vi "GeneratePointsForStage.vi"(8 "error in (no error)":errorcluster, 10 "Point Spacing":i32=20, 11 "Rotated Rect":T1(array[cluster])) -> (0 "error out":errorcluster, 3 "PointsInRotatedRect":cluster{"X":i32, "Y":i32}[](array[cluster]))   [LabVIEW 2017]
doc: "Use this template to build a VI to use as a subVI."
uses:
  <vilib>/Analysis/geometry.llb/Point in Polygon Position.ctl
  <vilib>/Analysis/coordinate.llb/2D Cartesian Coordinate Shift (Array).vi
  <vilib>/Analysis/coordinate.llb/2D Cartesian Coordinate Rotation (Array).vi
  <vilib>/Analysis/geometry.llb/Point in Polygon (Scalar).vi
  <vilib>/Analysis/NI_AAL_Geometry.lvlib
  <vilib>/Analysis/NI_AALPro.lvlib
panel:
  out "point":cluster{"x":i16, "y":i16}={"x"=1139, "y"=846}
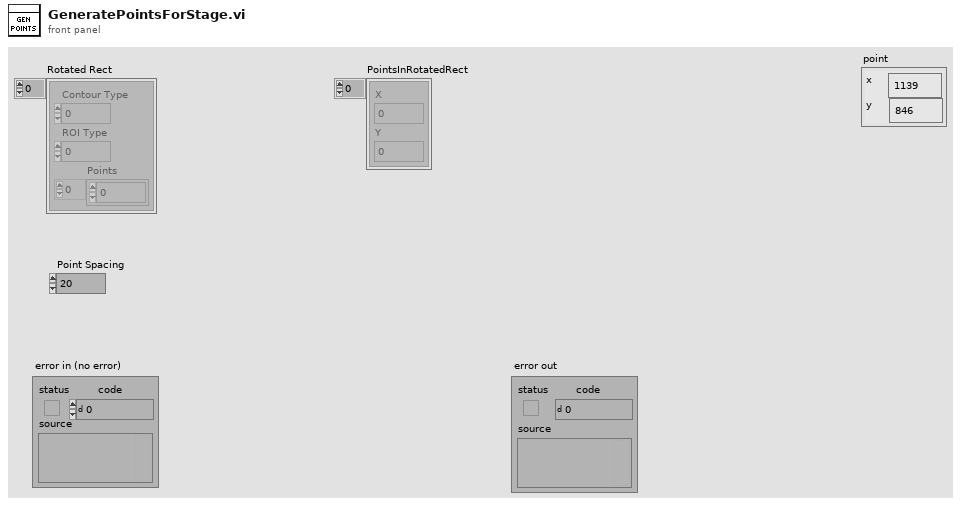
[diagram p1: front panel]
types:
  T1 = cluster{"Contour Type":u32, "ROI Type":u32, "Points":i32[]}[]
  T2 = cluster{"left":i16, "top":i16, "right":i16, "bottom":i16}
  T3 = cluster{"Contour Type":u32, "ROI Type":u32, "Points":i32[]}
  T4 = typedef "NI_AAL_Geometry.lvlib/Point in Polygon Position.ctl" = u16
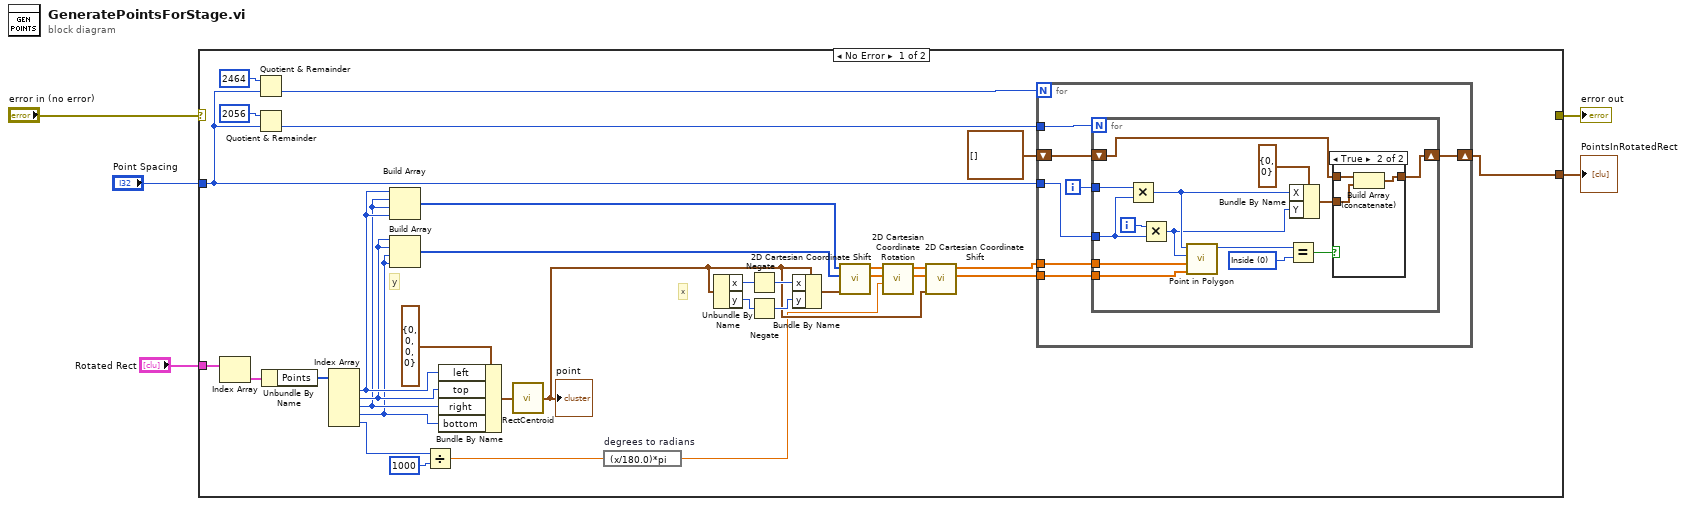
[diagram p0: block diagram]
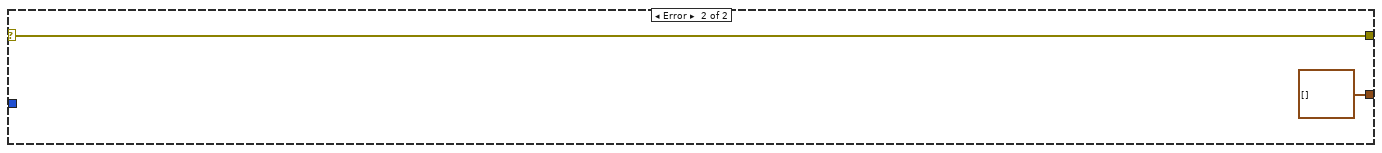
[diagram p3: hidden frame]
diagram:
  n1 = case shown="No Error" "error in (no error)" {
    selector: "error in (no error)" -> [_ w66]
    tunnel: [_ w66] -> w4
    tunnel: "Rotated Rect" -> [w8 _]
    tunnel: [w6 cluster{"X":i32, "Y":i32}[] []] -> w2
    tunnel: "Point Spacing" -> [w7 _]
    frame No Error {
      # "y"
      # "x"
      n2 = Index Array(array=w8) -> (element=w23:T3)  [unwired: 1 in]
      n3 = Quotient & Remainder(x=2464, y=w7) -> (floor(x/y)=w39:i32)  [unwired: 1 out]
      n4 = Quotient & Remainder(x=2056, y=w7) -> (floor(x/y)=w38:i32)  [unwired: 1 out]
      n5 = Unbundle By Name(w23) -> ("Points"=w22:i32[])
      n6 = Index Array(array=w22) -> (element #1=w12:i32, element #2=w11:i32, element #3=w10:i32, element #4=w9:i32, element #5=w21:i32)  [unwired: 5 in]
      n7 = Build Array(w12, w10, w10, w12) -> (w32:i32[])
      n8 = Build Array(w11, w11, w9, w9) -> (w31:i32[])
      n9 = Divide(x=w21, y=1000) -> (x/y=w19:dbl)
      n10 = Bundle By Name(cluster=T2 {"left"=0, "top"=0, "right"=0, "bottom"=0} ("rect"), "left"=w12, "top"=w11, "right"=w10, "bottom"=w9) -> (w33:T2)
      n11 = call <vilib>:"RectCentroid.vi"("rect"=w33) -> ("point"=w16:cluster{"x":i16, "y":i16})
      "point" <- w16
      n12 = expression code="(x/180.0)*pi" "degrees to radians"(w19) -> (w13:dbl)
      n13 = Unbundle By Name(w16) -> ("x"=w30:i16, "y"=w29:i16)
      n14 = Negate(x=w30) -> (-x=w28:i16)
      n15 = Negate(x=w29) -> (-x=w27:i16)
      n16 = Bundle By Name(cluster=w16, "x"=w28, "y"=w27) -> (w26:cluster{"x":i16, "y":i16})
      n17 = call-poly <vilib>:"2D Cartesian Coordinate Shift.vi"("shift"=w26, "Y"=w31, "X"=w32) -> ("Y Out"=w24:dbl[], "X Out"=w25:dbl[])  [unwired: 6 in, 1 out]
      n18 = call-poly <vilib>:"2D Cartesian Coordinate Rotation.vi"("theta"=w13, "Y"=w24, "X"=w25) -> ("Y Out"=w17:dbl[], "X Out"=w18:dbl[])  [unwired: 6 in, 1 out]
      n19 = call-poly <vilib>:"2D Cartesian Coordinate Shift.vi"("shift"=w16, "Y"=w17, "X"=w18) -> ("Y Out"=w14:dbl[], "X Out"=w15:dbl[])  [unwired: 6 in, 1 out]
      n20 = for {
        N: w39 -> [_]
        tunnel: w38 -> [w46]
        tunnel: w7 -> [w44]
        shift-right: [w40] -> w6
        shift-left: cluster{"X":i32, "Y":i32}[] [] -> [w43]
        tunnel: w15 -> [w42]
        tunnel: w14 -> [w41]
        i -> [w45]
        n21 = for {
          N: w46 -> [_]
          tunnel: w45 -> [w57]
          tunnel: w44 -> [w59]
          shift-right: [w55] -> w40
          shift-left: w43 -> [w54]
          tunnel: w42 -> [w53]
          tunnel: w41 -> [w52]
          i -> [w58]
          w48 = T4 0 items=["Inside", "On Boundary", "Outside"] ("y")
          n22 = Multiply(x=w57, y=w59) -> (x*y=w51:i32)
          n23 = Multiply(x=w58, y=w59) -> (x*y=w50:i32)
          n24 = call-poly <vilib>:"Point in Polygon.vi"("Polygon Y"=w52, "Polygon X"=w53, "y"=w50, "x"=w51) -> ("position"=w49:T4)  [unwired: 6 in, 1 out]
          n25 = Equal?(x=w49, y=w48) -> (x = y?=w47:bool)
          n26 = Bundle By Name(cluster=cluster{"X":i32, "Y":i32} {"X"=0, "Y"=0} ("Point Coordinates"), "X"=w51, "Y"=w50) -> (w56:cluster{"X":i32, "Y":i32})
          n27 = case shown="True" w47 {
            tunnel: w56 -> [_ w64]
            tunnel: [w61 w63] -> w55
            tunnel: w54 -> [w61 w62]
            frame False {
            }
            frame True {
              n28 = Build Array (concatenate)(w62, w64) -> (w63:cluster{"X":i32, "Y":i32}[])
            }
          }
        }
      }
    }
    frame Error {
    }
  }
  "error out" <- w4
  "PointsInRotatedRect" <- w2
